vi "display_michelle_visjitter_stopadded.vi"() -> ()   [LabVIEW 2019]
uses:
  <vilib>/Analysis/Matrix/Datatypes/RealMatrix.ctl
  <vilib>/Utility/file.llb/Write Delimited Spreadsheet (DBL).vi
  <vilib>/Analysis/Matrix/NI_Matrix.lvlib
panel:
  out "maxITI":dbl
  out "minITI":dbl
  out "lambda":dbl
  out "goEXP":dbl
  out "TimeOutCounter":i32
  out "ElapsedTime_M":dbl
  out "IMG_Contrast":dbl
  out "CurrentTrial":u32=1
  out "Jitter":dbl
  out "BaseITI":dbl
  out "VisStimDuration":dbl
  in  "Stop":bool
  out "Num trials":u32=204
  out "ISI Time":dbl
  out "Stim TS":dbl
  out "Output":dbl[][](array[numeric])
  out "Output frame":T1
  out "Array temp1":T1
  out "Elapsed Time":dbl
  out "Display":bool=TRUE
  out "Trial":u32=1
  out "reward":dbl[](array[numeric])
  out "stim_id":dbl[](array[numeric])
  out "stim_loaded":dbl
  out "Timings":dbl[](array[numeric])
  out "Stimuli Loaded?":bool
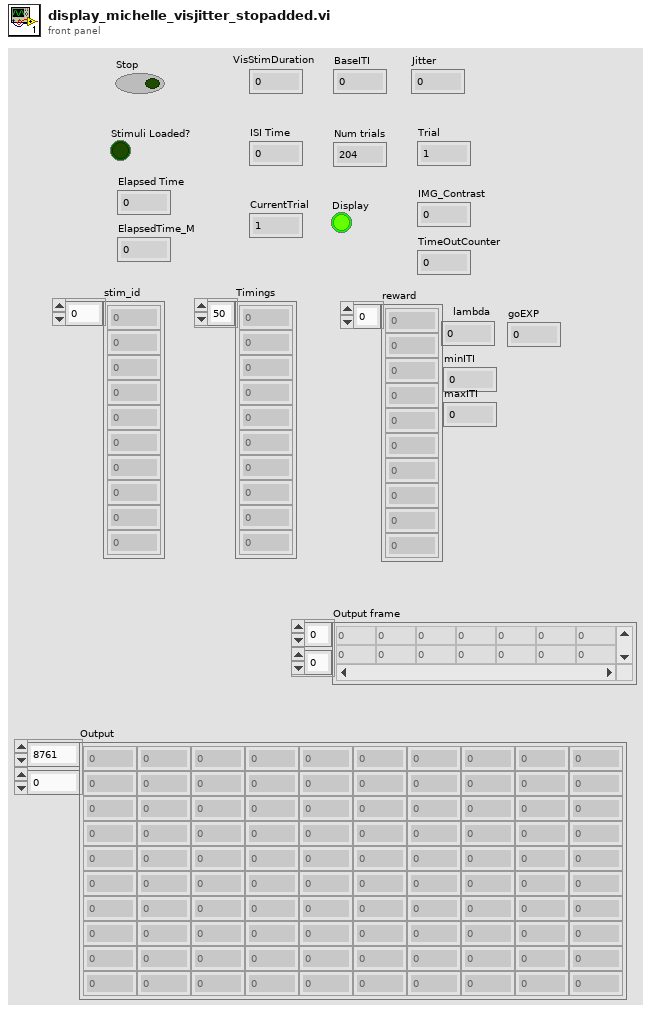
[diagram p1: front panel]
types:
  T1 = typedef "NI_Matrix.lvlib/RealMatrix.ctl" = dbl[][]
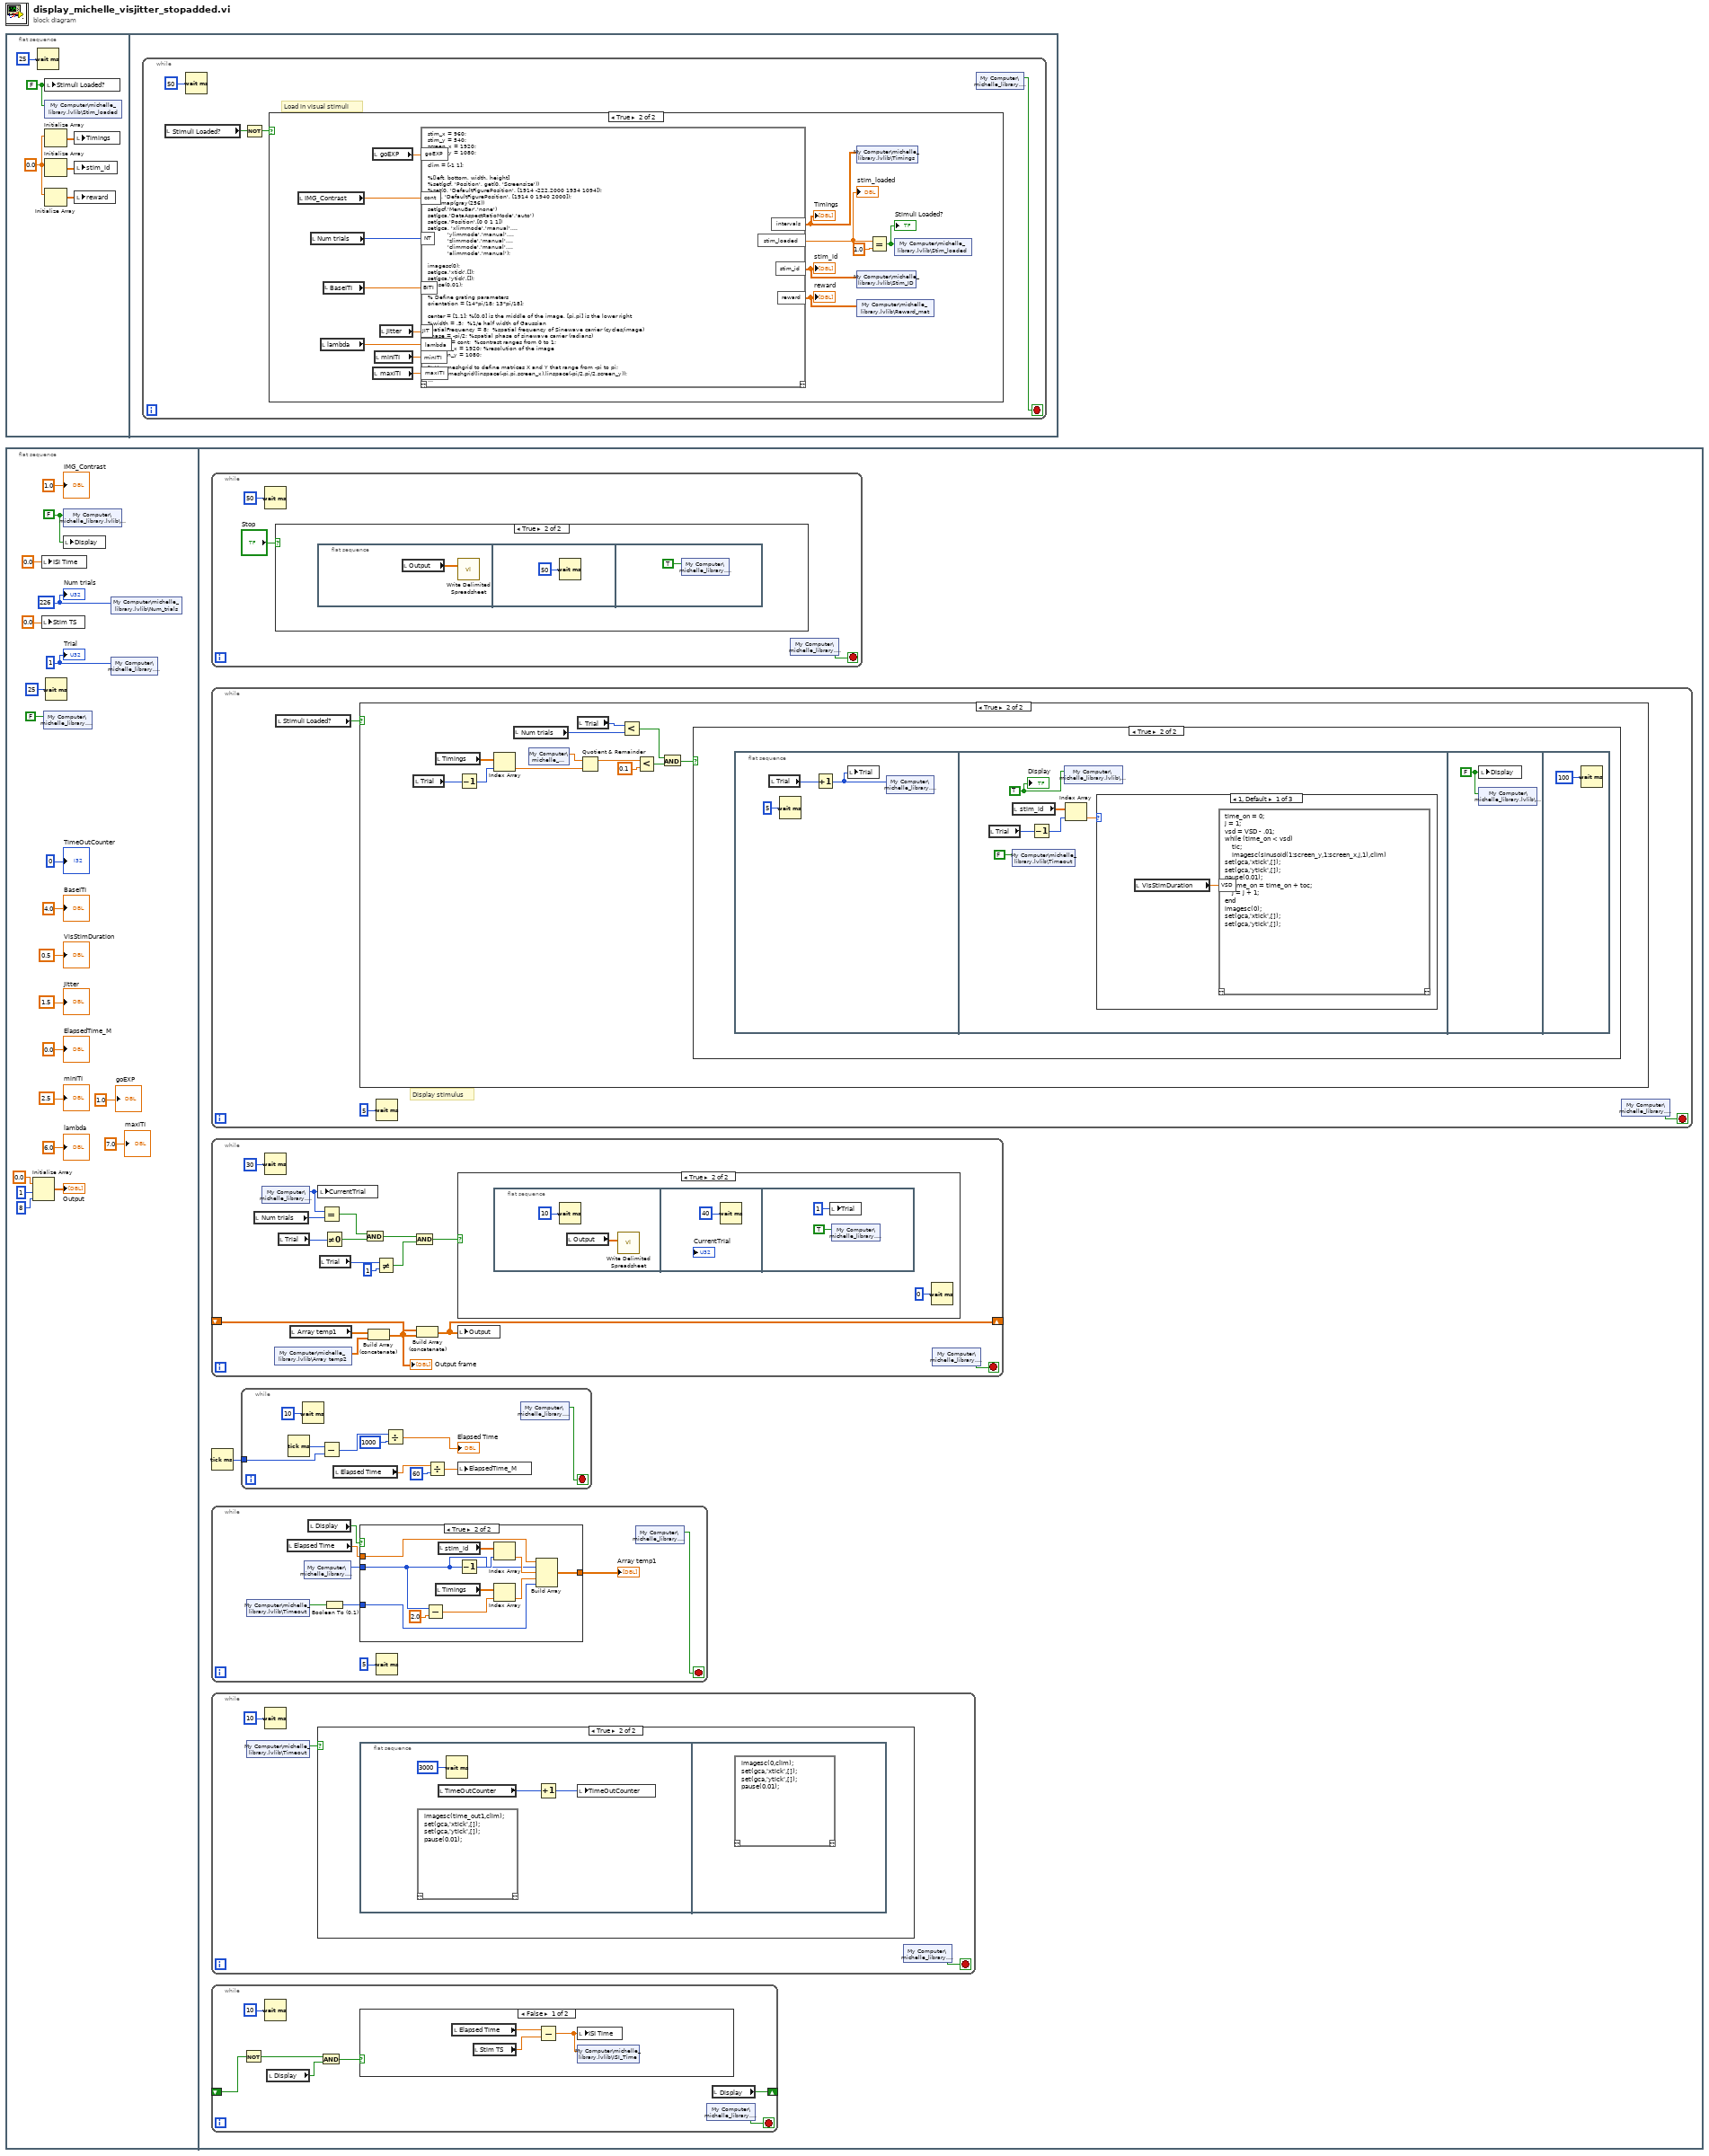
[diagram p0: block diagram]
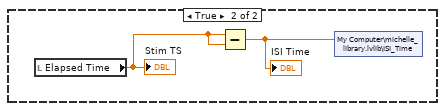
[diagram p5: hidden frame]
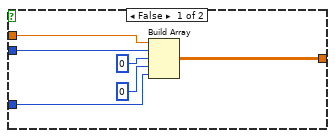
[diagram p6: hidden frame]
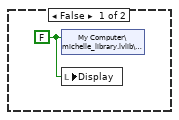
[diagram p9: hidden frame]
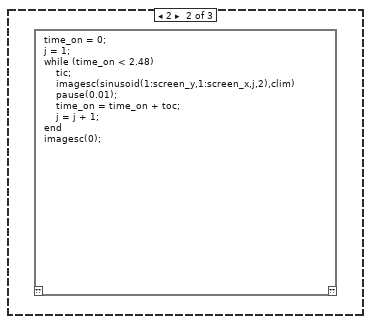
[diagram p10: hidden frame]
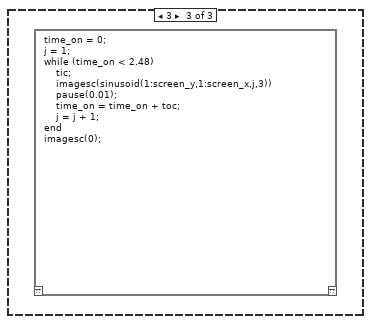
[diagram p11: hidden frame]
diagram:
  n1 = flat-sequence {
    frame #0 {
      w3 = 0.0 ("element")
      w1 = FALSE ("Stimuli Loaded?")
      n2 = Wait (ms)(milliseconds to wait=u32 25) -> ()  [unwired: 1 out]
      n3 = local write "Stimuli Loaded?"(w1) -> ()
      n4 = shared-variable "My Computer\\michelle_library.lvlib\\Stim_loaded"(w1) -> ()  [unwired: 1 in, 1 out]
      n5 = Initialize Array(w3) -> (w5:dbl[])  [unwired: 1 in]
      n6 = Initialize Array(w3) -> (w4:dbl[])  [unwired: 1 in]
      n7 = Initialize Array(w3) -> (w2:dbl[])  [unwired: 1 in]
      n8 = local write "Timings"(w5) -> ()
      n9 = local write "stim_id"(w4) -> ()
      n10 = local write "reward"(w2) -> ()
    }
    frame #1 {
      n11 = while {
        stop <- w9 stop-if-true
        # "Load in visual stimuli"
        n12 = local read "Stimuli Loaded?"() -> (w8:bool)
        n13 = Wait (ms)(milliseconds to wait=u32 50) -> ()  [unwired: 1 out]
        n14 = Not(x=w8) -> (.not. x?=w7:bool)
        n15 = case shown="True" w7 {
          frame False {
          }
          frame True {
            n16 = local read "IMG_Contrast"() -> (w15:dbl)
            n17 = local read "Num trials"() -> (w18:u32)
            n18 = local read "lambda"() -> (w13:dbl)
            n19 = local read "BaseITI"() -> (w17:dbl)
            n20 = local read "goEXP"() -> (w14:dbl)
            n21 = local read "maxITI"() -> (w11:dbl)
            n22 = local read "minITI"() -> (w12:dbl)
            n23 = local read "Jitter"() -> (w16:dbl)
            n24 = script code="stim_x = 960;\nstim_y = 540;\nscreen_x = 1920;\nscreen_y = 1080;\n\nclim = [-1 1];\n\n%[left, bottom, width, height]\n%set(gcf, 'Position', get(0, 'Screensize'))\n%set(0, 'DefaultFigurePosition', [1914 -222.2000 1934 1094]);\nset(0, 'DefaultFigurePosition', [1914 0 1940 2000]);\ncolormap(gray(256))\nset(gcf,'MenuBar','none')\nset(gca,'DataAspectRatioMode','auto')\nset(gca,'Position',[0 0 1 1])\nset(gca, 'xlimmode','manual',...\n           'ylimmode','manual',...\n           'zlimmode','manual',...\n           'climmode','manual',...\n           'alimmode','manual');\n\nimagesc(0);\nset(gca,'xtick',[]);\nset(gca,'ytick',[]);\npause(0.01);\n\n% Define grating parameters\norientation = [14*pi/18; 13*pi/18];\n\ncenter = [1,1]; %[0,0] is the middle of the image, [pi,pi] is the lower right\n%width = .5;  %1/e half width of Gaussian\nspatialFrequency = 8;  %spatial frequency of Sinewave carrier (cycles/image)\nphase = -pi/2; %spatial phase of sinewave carrier (radians)\ncontrast = cont;  %contrast ranges from 0 to 1;\n%screen_x = 1920; %resolution of the image  \n%screen_y = 1080;\n\n% Use meshgrid to define matrices X and Y that range from -pi to pi;\n[X,Y] = meshgrid(linspace(-pi,pi,screen_x),linspace(-pi/2,pi/2,screen_y));\n\nsinusoid = zeros(screen_y,screen_x,150,2);\ntime_out1 = ones(screen_y,screen_x)*-1;\ntime_out2 = zeros(screen_y,screen_x);\n%time_out(1,1) = 1;\n% Set up individual 4-d matrices (x, y, time, orientation) for movies of the drifting gratings at each\n% orientation\nfor j = 1:length(orientation)                                                            % Phase increase number here\n    ramp(1:screen_y,1:screen_x,j) = cos(orientation(j))*(X-center(1)) + sin(orientation(j))*(Y-center(2));     %  |\n    for i = 1:150 %Sets the number of frames to define gratings for                   V\n       sinusoid(1:screen_y,1:screen_x,i,j) = contrast*sin(spatialFrequency*ramp(1:screen_y,1:screen_x,j)-...\n           (phase+(2*pi*(i-1)*(-30)/360))); %Number before '/360' sets the phase increase\n    end\nend\n\n%%  To be run of not using exponential\n%intervals = [ones(1,41)*10 ones(1,41)*11 ones(1,41)*12 ones(1,41)*13 ones(1,40)*14];\nif goEXP < 1\njit = JIT;\njitter = rand(1,NT);\njitter = 2*jit*(jitter- .5);\nITIbase = BITI;\nintervals = [ones(1,NT)*ITIbase];\nintervals = intervals + jitter;\nelseif goEXP > 0\n            intervals = exponentialITI(1/lambda ,minITI ,maxITI , NT);\nend\n%%\nstim_id = [ones(1,NT)*1];\n%reward = [ones(1,87)*1 ones(1,15)*0 ones(1,87)*1 ones(1,15)*0];\nreward = [ones(1,NT)*1];\n\nrand_idx1 = randperm(NT);\nrand_idx2 = randperm(NT);\nintervals = intervals(rand_idx2);\nstim_id = stim_id(rand_idx2);\nreward = reward(rand_idx2);\n\nstim_loaded = 1;" ("Script Node")("NT"=w18, "BITI"=w17, "JIT"=w16, "cont"=w15, "goEXP"=w14, "minITI"=w12, "maxITI"=w11, "lambda"=w13) -> ("stim_loaded"=w24:dbl, "intervals"=w19:dbl[], "stim_id"=w20:dbl[], "reward"=w22:dbl[])  [unwired: 1 in, 1 out]
            "stim_loaded" <- w24
            "Timings" <- w19
            "stim_id" <- w20
            "reward" <- w22
            n25 = shared-variable "My Computer\\michelle_library.lvlib\\Timings"(w19) -> ()  [unwired: 1 in, 1 out]
            n26 = shared-variable "My Computer\\michelle_library.lvlib\\Stim_ID"(w20) -> ()  [unwired: 1 in, 1 out]
            n27 = shared-variable "My Computer\\michelle_library.lvlib\\Reward_mat"(w22) -> ()  [unwired: 1 in, 1 out]
            n28 = Equal?(x=w24, y=1.0) -> (x = y?=w21:bool)
            "Stimuli Loaded?" <- w21
            n29 = shared-variable "My Computer\\michelle_library.lvlib\\Stim_loaded"(w21) -> ()  [unwired: 1 in, 1 out]
          }
        }
        n30 = shared-variable "My Computer\\michelle_library.lvlib\\Stop"() -> (w9:bool)  [unwired: 1 in, 1 out]
      }
    }
  }
  n31 = flat-sequence {
    frame #0 {
      w37 = u32 226
      w43 = FALSE ("Display")
      w45 = u32 1 ("Trial")
      n32 = Initialize Array(0.0 ("element"), 1 ("dimension size"), 8 ("dimension size")) -> (→"Output":dbl[][])
      n33 = local write "ISI Time"(0.0 ("ISI Time")) -> ()
      n34 = local write "Stim TS"(0.0 ("Stim TS")) -> ()
      n35 = shared-variable "My Computer\\michelle_library.lvlib\\Stop"(FALSE ("Stop")) -> ()  [unwired: 1 in, 1 out]
      n36 = Wait (ms)(milliseconds to wait=u32 25) -> ()  [unwired: 1 out]
      n37 = shared-variable "My Computer\\michelle_library.lvlib\\Display"(w43) -> ()  [unwired: 1 in, 1 out]
      n38 = local write "Display"(w43) -> ()
      n39 = shared-variable "My Computer\\michelle_library.lvlib\\Num_trials"(w37) -> ()  [unwired: 1 in, 1 out]
      n40 = shared-variable "My Computer\\michelle_library.lvlib\\Trial"(w45) -> ()  [unwired: 1 in, 1 out]
      "Trial" <- w45
      "Num trials" <- w37
      "VisStimDuration" <- 0.5
      "BaseITI" <- 4.0
      "Jitter" <- 1.5
      "IMG_Contrast" <- 1.0
      "ElapsedTime_M" <- 0.0
      "TimeOutCounter" <- 0
      "goEXP" <- 1.0
      "lambda" <- 6.0
      "minITI" <- 2.5
      "maxITI" <- 7.0
    }
    frame #1 {
      n41 = while {
        stop <- w49 stop-if-true
        n42 = Wait (ms)(milliseconds to wait=50) -> ()  [unwired: 1 out]
        n43 = case shown="True" "Stop" {
          frame False {
          }
          frame True {
            n44 = flat-sequence {
              frame #0 {
                n45 = local read "Output"() -> (w50:dbl[][])
                n46 = call-poly <vilib>:"Write Delimited Spreadsheet.vi"("2D data"=w50) -> ()  [unwired: 13 in, 2 out]
              }
              frame #1 {
                n47 = Wait (ms)(milliseconds to wait=50) -> ()  [unwired: 1 out]
              }
              frame #2 {
                n48 = shared-variable "My Computer\\michelle_library.lvlib\\Stop"(TRUE) -> ()  [unwired: 1 in, 1 out]
              }
            }
          }
        }
        n49 = shared-variable "My Computer\\michelle_library.lvlib\\Stop"() -> (w49:bool)  [unwired: 1 in, 1 out]
      }
      n50 = while {
        stop <- w130 stop-if-true
        # "Display stimulus"
        n51 = local read "Stimuli Loaded?"() -> (w129:bool)
        n52 = case shown="True" w129 {
          frame False {
          }
          frame True {
            n53 = local read "Trial"() -> (w132:u32)
            n54 = local read "Timings"() -> (w141:dbl[])
            n55 = Decrement(x=w132) -> (x-1=w133:u32)
            n56 = Index Array(array=w141, index=w133) -> (element=w140:dbl)
            n57 = local read "Num trials"() -> (w136:u32)
            n58 = shared-variable "My Computer\\michelle_library.lvlib\\ISI"() -> (w135:dbl)  [unwired: 1 in, 1 out]
            n59 = local read "Trial"() -> (w139:u32)
            n60 = Quotient & Remainder(x=w135, y=w140) -> (x-y*floor(x/y)=w143:dbl)  [unwired: 1 out]
            n61 = Less?(x=w139, y=w136) -> (x < y?=w138:bool)
            n62 = Less?(x=w143, y=0.1) -> (x < y?=w137:bool)
            n63 = And(x=w138, y=w137) -> (x .and. y?=w134:bool)
            n64 = case shown="True" w134 {
              frame False {
                w144 = FALSE ("Display")
                n65 = shared-variable "My Computer\\michelle_library.lvlib\\Display"(w144) -> ()  [unwired: 1 in, 1 out]
                n66 = local write "Display"(w144) -> ()
              }
              frame True {
                n67 = flat-sequence {
                  frame #0 {
                    n68 = local read "Trial"() -> (w147:u32)
                    n69 = Wait (ms)(milliseconds to wait=u32 5) -> ()  [unwired: 1 out]
                    n70 = Increment(x=w147) -> (x+1=w146:u32)
                    n71 = local write "Trial"(w146) -> ()
                    n72 = shared-variable "My Computer\\michelle_library.lvlib\\Trial"(w146) -> ()  [unwired: 1 in, 1 out]
                  }
                  frame #1 {
                    w152 = TRUE ("Boolean")
                    n73 = local read "Trial"() -> (w150:u32)
                    n74 = local read "stim_id"() -> (w153:dbl[])
                    n75 = shared-variable "My Computer\\michelle_library.lvlib\\Timeout"(FALSE) -> ()  [unwired: 1 in, 1 out]
                    n76 = Decrement(x=w150) -> (x-1=w149:u32)
                    n77 = shared-variable "My Computer\\michelle_library.lvlib\\Display"(w152) -> ()  [unwired: 1 in, 1 out]
                    n78 = Index Array(array=w153, index=w149) -> (element=w151:dbl)
                    n79 = case shown="1, Default" w151 {
                      frame 1, Default {
                        n80 = local read "VisStimDuration"() -> (w154:dbl)
                        n81 = script code="time_on = 0;\nj = 1;\nvsd = VSD - .01;\nwhile (time_on < vsd)\n    tic;\n    imagesc(sinusoid(1:screen_y,1:screen_x,j,1),clim)\nset(gca,'xtick',[]);\nset(gca,'ytick',[]);    \npause(0.01);\n    time_on = time_on + toc;\n    j = j + 1;\nend\nimagesc(0);\nset(gca,'xtick',[]);\nset(gca,'ytick',[]);"("VSD"=w154) -> ()  [unwired: 1 in, 1 out]
                      }
                      frame 2 {
                        n82 = script code="time_on = 0;\nj = 1;\nwhile (time_on < 2.48)\n    tic;\n    imagesc(sinusoid(1:screen_y,1:screen_x,j,2),clim)\n    pause(0.01);\n    time_on = time_on + toc;\n    j = j + 1;\nend\nimagesc(0);"() -> ()  [unwired: 1 in, 1 out]
                      }
                      frame 3 {
                        n83 = script code="time_on = 0;\nj = 1;\nwhile (time_on < 2.48)\n    tic;\n    imagesc(sinusoid(1:screen_y,1:screen_x,j,3))\n    pause(0.01);\n    time_on = time_on + toc;\n    j = j + 1;\nend\nimagesc(0);"() -> ()  [unwired: 1 in, 1 out]
                      }
                    }
                    "Display" <- w152
                  }
                  frame #2 {
                    w155 = FALSE ("Display")
                    n84 = local write "Display"(w155) -> ()
                    n85 = shared-variable "My Computer\\michelle_library.lvlib\\Display"(w155) -> ()  [unwired: 1 in, 1 out]
                  }
                  frame #3 {
                    n86 = Wait (ms)(milliseconds to wait=u32 100) -> ()  [unwired: 1 out]
                  }
                }
              }
            }
          }
        }
        n87 = Wait (ms)(milliseconds to wait=u32 5) -> ()  [unwired: 1 out]
        n88 = shared-variable "My Computer\\michelle_library.lvlib\\Stop"() -> (w130:bool)  [unwired: 1 in, 1 out]
      }
      n89 = while {
        shift-right: [w119] -> _
        shift-left: _ -> [w120]
        stop <- w122 stop-if-true
        n90 = local read "Num trials"() -> (w115:u32)
        n91 = shared-variable "My Computer\\michelle_library.lvlib\\Trial"() -> (w106:u32)  [unwired: 1 in, 1 out]
        n92 = Wait (ms)(milliseconds to wait=u32 30) -> ()  [unwired: 1 out]
        n93 = shared-variable "My Computer\\michelle_library.lvlib\\Array temp2"() -> (w117:dbl[][])  [unwired: 1 in, 1 out]
        n94 = local read "Trial"() -> (w113:u32)
        n95 = local read "Array temp1"() -> (w118:T1)
        n96 = local write "CurrentTrial"(w106) -> ()
        n97 = local read "Trial"() -> (w112:u32)
        n98 = Equal?(x=w106, y=w115) -> (x = y?=w114:bool)
        n99 = Not Equal To 0?(x=w113) -> (x != 0?=w109:bool)
        n100 = And(x=w114, y=w109) -> (x .and. y?=w107:bool)
        n101 = Build Array (concatenate)(w118, w117) -> (w116:T1)
        "Output frame" <- w116
        n102 = Not Equal?(x=w112, y=1) -> (x != y?=w111:bool)
        n103 = And(x=w107, y=w111) -> (x .and. y?=w108:bool)
        n104 = Build Array (concatenate) ("Build Matrix")(w120, w116) -> (w119:T1)
        n105 = case shown="True" w108 {
          frame False {
          }
          frame True {
            n106 = flat-sequence {
              frame #0 {
                n107 = Wait (ms)(milliseconds to wait=u32 10) -> ()  [unwired: 1 out]
                n108 = local read "Output"() -> (w125:dbl[][])
                n109 = call-poly <vilib>:"Write Delimited Spreadsheet.vi"("2D data"=w125) -> ()  [unwired: 13 in, 2 out]
              }
              frame #1 {
                n110 = Wait (ms)(milliseconds to wait=u32 40) -> ()  [unwired: 1 out]
              }
              frame #2 {
                n111 = local write "Trial"(1) -> ()
                n112 = shared-variable "My Computer\\michelle_library.lvlib\\Stop"(TRUE) -> ()  [unwired: 1 in, 1 out]
              }
            }
            n113 = Wait (ms)(milliseconds to wait=0) -> ()  [unwired: 1 out]
          }
        }
        n114 = local write "Output"(w119) -> ()
        n115 = shared-variable "My Computer\\michelle_library.lvlib\\Stop"() -> (w122:bool)  [unwired: 1 in, 1 out]
      }
      n116 = Tick Count (ms)() -> (millisecond timer value=w46:u32)
      n117 = while {
        stop <- w73 stop-if-true
        n118 = shared-variable "My Computer\\michelle_library.lvlib\\Timeout"() -> (w71:bool)  [unwired: 1 in, 1 out]
        n119 = local read "Elapsed Time"() -> (w77:dbl)
        n120 = shared-variable "My Computer\\michelle_library.lvlib\\Trial"() -> (w75:u32)  [unwired: 1 in, 1 out]
        n121 = local read "Display"() -> (w74:bool)
        n122 = Boolean To (0,1)(Boolean=w71) -> (0, 1=w72:i16)
        n123 = case shown="True" w74 {
          tunnel: w75 -> [w83 w86]
          tunnel: w77 -> [w84 w93]
          tunnel: [w82 w94] -> w76
          tunnel: w72 -> [w79 w88]
          frame False {
            n124 = Build Array(w84, w83, u32 0 ("milliseconds to wait"), 0, w79) -> (w82:T1)
          }
          frame True {
            n125 = Subtract(x=w86, y=2.0) -> (x-y=w85:dbl)
            n126 = local read "Timings"() -> (w91:dbl[])
            n127 = local read "stim_id"() -> (w95:dbl[])
            n128 = Decrement(x=w86) -> (x-1=w90:u32)
            n129 = Index Array(array=w95, index=w90) -> (element=w92:dbl)
            n130 = Index Array(array=w91, index=w85) -> (element=w89:dbl)
            n131 = Build Array(w93, w86, w92, w89, w88) -> (w94:T1)
          }
        }
        "Array temp1" <- w76
        n132 = Wait (ms)(milliseconds to wait=u32 5) -> ()  [unwired: 1 out]
        n133 = shared-variable "My Computer\\michelle_library.lvlib\\Stop"() -> (w73:bool)  [unwired: 1 in, 1 out]
      }
      n134 = while {
        stop <- w55 stop-if-true
        n135 = shared-variable "My Computer\\michelle_library.lvlib\\Timeout"() -> (w53:bool)  [unwired: 1 in, 1 out]
        n136 = Wait (ms)(milliseconds to wait=u32 10) -> ()  [unwired: 1 out]
        n137 = case shown="True" w53 {
          frame False {
          }
          frame True {
            n138 = flat-sequence {
              frame #0 {
                n139 = script code="imagesc(time_out1,clim);\nset(gca,'xtick',[]);\nset(gca,'ytick',[]);\npause(0.01);"() -> ()  [unwired: 1 in, 1 out]
                n140 = local read "TimeOutCounter"() -> (w57:i32)
                n141 = Wait (ms)(milliseconds to wait=u32 3000) -> ()  [unwired: 1 out]
                n142 = Increment(x=w57) -> (x+1=w56:i32)
                n143 = local write "TimeOutCounter"(w56) -> ()
              }
              frame #1 {
                n144 = script code="imagesc(0,clim);\nset(gca,'xtick',[]);\nset(gca,'ytick',[]);\npause(0.01);"() -> ()  [unwired: 1 in, 1 out]
              }
            }
          }
        }
        n145 = shared-variable "My Computer\\michelle_library.lvlib\\Stop"() -> (w55:bool)  [unwired: 1 in, 1 out]
      }
      n146 = while {
        shift-right: [w63] -> _
        shift-left: _ -> [w62]
        stop <- w65 stop-if-true
        n147 = Not(x=w62) -> (.not. x?=w61:bool)
        n148 = Wait (ms)(milliseconds to wait=u32 10) -> ()  [unwired: 1 out]
        n149 = local read "Display"() -> (w60:bool)
        n150 = And(x=w61, y=w60) -> (x .and. y?=w59:bool)
        n151 = case shown="False" w59 {
          frame False {
            n152 = local read "Elapsed Time"() -> (w66:dbl)
            n153 = local read "Stim TS"() -> (w68:dbl)
            n154 = Subtract(x=w66, y=w68) -> (x-y=w67:dbl)
            n155 = local write "ISI Time"(w67) -> ()
            n156 = shared-variable "My Computer\\michelle_library.lvlib\\ISI_Time"(w67) -> ()  [unwired: 1 in, 1 out]
          }
          frame True {
            n157 = local read "Elapsed Time"() -> (w69:dbl)
            "Stim TS" <- w69
            n158 = Subtract(x=w69, y=w69) -> (x-y=w70:dbl)
            "ISI Time" <- w70
            n159 = shared-variable "My Computer\\michelle_library.lvlib\\ISI_Time"(w70) -> ()  [unwired: 1 in, 1 out]
          }
        }
        n160 = shared-variable "My Computer\\michelle_library.lvlib\\Stop"() -> (w65:bool)  [unwired: 1 in, 1 out]
        n161 = local read "Display"() -> (w63:bool)
      }
      n162 = while {
        tunnel: w46 -> [w102]
        stop <- w99 stop-if-true
        n163 = Tick Count (ms)() -> (millisecond timer value=w103:u32)
        n164 = Wait (ms)(milliseconds to wait=u32 10) -> ()  [unwired: 1 out]
        n165 = Subtract(x=w103, y=w102) -> (x-y=w100:u32)
        n166 = local read "Elapsed Time"() -> (w96:dbl)
        n167 = Divide(x=w100, y=u32 1000) -> (x/y=→"Elapsed Time":dbl)
        n168 = Divide(x=w96, y=60) -> (x/y=w98:dbl)
        n169 = local write "ElapsedTime_M"(w98) -> ()
        n170 = shared-variable "My Computer\\michelle_library.lvlib\\Stop"() -> (w99:bool)  [unwired: 1 in, 1 out]
      }
    }
  }
